vi "LUCS001RT_GPS_Processor.vi"(6 "SinchronizationReferences":T1, 7 "FPGA VI Reference Out":T3, 8 "error in":errorcluster, 11 "GPS DataIn":T4 {"UTC Valid" items=["UTC not valid", "Valid Time of Week", "Valid Week Number", "NA", "Valid UTC"]; "CAcc" format="%.0f°"; "Heading(2-D)" format="%0.6f°"; "GSpeed(2-D)" format="%.0f cm/s"; "Speed(3-D)" format="%.0f cm/s"; "NED_DNvsty" format="%.0f cm/s"; "NED_Evsty" format="%.0f cm/s"; "NED_NVsty" format="%.0f cm/s"; "Sacc" format="%.0f cm/s"; "ECEF_Z_Vlsty" format="%.0f cm/s"; "ECEF_Y_Vlsty" format="%.0f cm/s"; "ECEF_X_Vlsty" format="%.0f cm/s"; "FixType" items=["No Fix", "Dead Reckoning Only", "2D-Fix", "3D-Fix", "GPS + Dead Reckoning", "Time Only Fix", "RESERVED"]; "Vacc" format="%.0f mm"; "Hacc" format="%.0f mm"; "HMSL" format="%d mm"; "HEIGHT" format="%.0f mm"; "LAT" format="%#.6f"; "LON" format="%#.6f"; "Waypoint:XTE" format="%#.2f"}) -> (0 "error out":errorcluster, 3 "GPS Data Out":T4 {"UTC Valid" items=["UTC not valid", "Valid Time of Week", "Valid Week Number", "NA", "Valid UTC"]; "CAcc" format="%.0f°"; "Heading(2-D)" format="%0.6f°"; "GSpeed(2-D)" format="%.0f cm/s"; "Speed(3-D)" format="%.0f cm/s"; "NED_DNvsty" format="%.0f cm/s"; "NED_Evsty" format="%.0f cm/s"; "NED_NVsty" format="%.0f cm/s"; "Sacc" format="%.0f cm/s"; "ECEF_Z_Vlsty" format="%.0f cm/s"; "ECEF_Y_Vlsty" format="%.0f cm/s"; "ECEF_X_Vlsty" format="%.0f cm/s"; "FixType" items=["No Fix", "Dead Reckoning Only", "2D-Fix", "3D-Fix", "GPS + Dead Reckoning", "Time Only Fix", "RESERVED"]; "Vacc" format="%.0f mm"; "Hacc" format="%.0f mm"; "HMSL" format="%d mm"; "HEIGHT" format="%.0f mm"; "LAT" format="%#.6f"; "LON" format="%#.6f"; "Waypoint:XTE" format="%#.2f"}, 4 "GPS.DataReceived":bool)   [LabVIEW 2024]
uses:
  LUCS001RT_GPS_Data.ctl
  cRIO Projects LV8.5/UAV/TypeDefs.llb/UMV_SinchronisationReferences.ctl
panel:
  # "WAYPOINT"
  # "CURRENT POSITION"
  # "WAYPOINT"
  # "CURRENT POSITION"
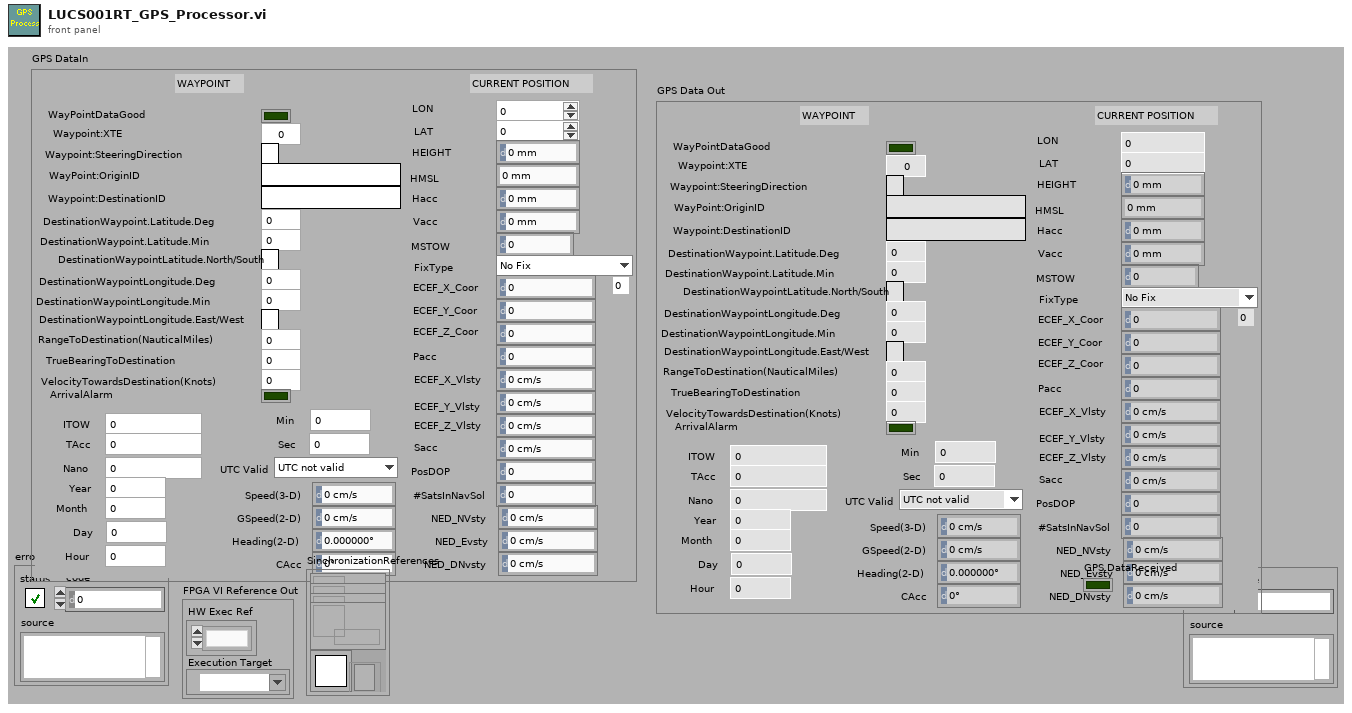
[diagram p1: front panel]
types:
  T1 = typedef "UMV_SinchronisationReferences.ctl" = cluster{"Notifier:LocalStop":refnum<notifier>, "Notifier:GlobalStop":refnum<notifier>, "RS232write":refnum<queue>, "RS232read":refnum<queue>, "RS232writeSynch":T2, "occurrence":refnum<k4>}
  T2 = typedef "Semaphore RefNum" = refnum<k1>
  T3 = cluster{"HW Exec Ref":refnum<k1>, "Execution Target":refnum<visa-resource-name>}
  T4 = typedef "LUCS001RT_GPS_Data.ctl" = cluster{"WayPointDataGood":bool, "Waypoint:XTE":dbl, "Waypoint:SteeringDirection":string, "WayPoint:OriginID":string, "Waypoint:DestinationID":string, "DestinationWaypoint.Latitude.Deg":i32, "DestinationWaypoint.Latitude.Min":dbl, "DestinationWaypointLatitude.North/South":string, "DestinationWaypointLongitude.Deg":i32, "DestinationWaypointLongitude.Min":dbl, "DestinationWaypointLongitude.East/West":string, "RangeToDestination(NauticalMiles)":dbl, "TrueBearingToDestination":dbl, "VelocityTowardsDestination(Knots)":dbl, "ArrivalAlarm":bool, "ITOW":u32, "TAcc":u32, "LON":dbl, "LAT":dbl, "HEIGHT":i32, "HMSL":i32, "Hacc":u32, "Vacc":u32, "MSTOW":u32, "FixType":u8, "ECEF_X_Coor":i32, "ECEF_Y_Coor":i32, "ECEF_Z_Coor":i32, "Pacc":u32, "ECEF_X_Vlsty":i32, "ECEF_Y_Vlsty":i32, "ECEF_Z_Vlsty":i32, "Sacc":u32, "PosDOP":u16, "#SatsInNavSol":u8, "NED_NVsty":i32, "NED_Evsty":i32, "NED_DNvsty":i32, "Speed(3-D)":u32, "GSpeed(2-D)":u32, "Heading(2-D)":dbl, "CAcc":u32, "Nano":i32, "Year":u16, "Month":u8, "Day":u8, "Hour":u8, "Min":u8, "Sec":u8, "UTC Valid":u8}
  T5 = typedef "LUCS001RT_GPS_Data.ctl" = cluster{"WayPointDataGood":bool, "Waypoint:XTE":dbl, "Waypoint:SteeringDirection":string, "WayPoint:OriginID":string, "Waypoint:DestinationID":string, "DestinationWaypoint.Latitude.Deg":i32, "DestinationWaypoint.Latitude.Min":dbl, "DestinationWaypointLatitude.North/South":string, "DestinationWaypointLongitude.Deg":i32, "DestinationWaypointLongitude.Min":dbl, "DestinationWaypointLongitude.East/West":string, "RangeToDestination(NauticalMiles)":dbl, "TrueBearingToDestination":dbl, "VelocityTowardsDestination(Knots)":dbl, "ArrivalAlarm":bool, "System.Year":dbl, "System.DayOfTehYear":dbl, "LON":dbl, "LAT":dbl, "HEIGHT":i32, "HMSL":i32, "Hacc":u32, "Vacc":u32, "MSTOW":u32, "FixType":u8, "ECEF_X_Coor":i32, "ECEF_Y_Coor":i32, "ECEF_Z_Coor":i32, "Pacc":u32, "ECEF_X_Vlsty":i32, "ECEF_Y_Vlsty":i32, "ECEF_Z_Vlsty":i32, "Sacc":u32, "PosDOP":u16, "#SatsInNavSol":u8}
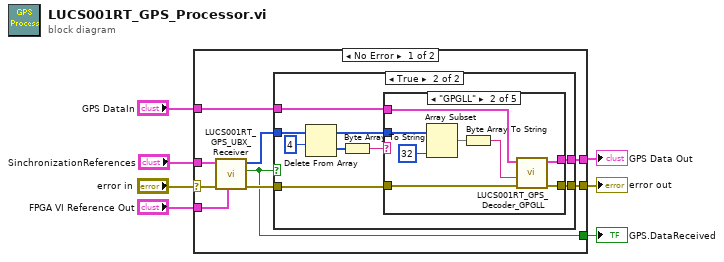
[diagram p0: block diagram]
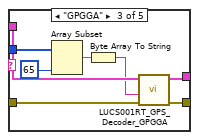
[diagram p4: hidden frame]
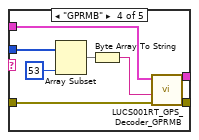
[diagram p5: hidden frame]
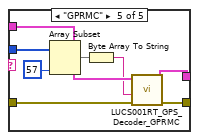
[diagram p6: hidden frame]
diagram:
  n1 = case shown="No Error" "error in" {
    selector: "error in" -> [w13 w62]
    tunnel: [w16 w62] -> w7
    tunnel: [w15 _] -> w6
    tunnel: "GPS DataIn" -> [w14 _]
    tunnel: "FPGA VI Reference Out" -> [w10 _]
    tunnel: [w9 _] -> w2
    tunnel: "SinchronizationReferences" -> [w11 _]
    frame No Error {
      n2 = call "LUCS001RT_GPS_UBX_Receiver.vi"("FPGA VI Reference In"=w10, "error in"=w13, "SinchronizationReferences"=w11) -> ("error out"=w12:errorcluster, "RX ArrayReady"=w9:bool, "GPS.TX.Message"=w8:u8[])  [unwired: 6 in]
      n3 = case shown="True" w9 {
        tunnel: [w18 w27] -> w16
        tunnel: [w17 w26] -> w15
        tunnel: w14 -> [w17 w25]
        tunnel: w12 -> [w18 w24]
        tunnel: w8 -> [_ w20]
        frame False {
        }
        frame True {
          n4 = Delete From Array(array=w20, length=4) -> (deleted portion=w19:u8[], array with subset deleted=w21:u8[])  [unwired: 1 in]
          n5 = Byte Array To String(unsigned byte array=w19) -> (string=w22:string)
          n6 = case shown="\"GPGLL\"" w22 {
            tunnel: w24 -> [w29 w33 w40 w50 w58]
            tunnel: [w29 w35 w43 w53 w61] -> w27
            tunnel: w25 -> [w28 w37 w45 w52 w60]
            tunnel: [w28 w36 w44 w51 w59] -> w26
            tunnel: w21 -> [_ w31 w39 w47 w55]
            frame Default {
            }
            frame "GPGLL" {
              n7 = Array Subset(array=w31, length=32 ("byte count")) -> (w30:u8[])  [unwired: 1 in]
              n8 = Byte Array To String(unsigned byte array=w30) -> (string=w32:string)
              n9 = call "LUCS001RT_GPS_Decoder_GPGLL.vi"("error in (no error)"=w33, "SerialData: GPGLL"=w32, "GPS Data In"=w37) -> ("error out"=w35:errorcluster, "GPS Data Out"=w36:T4)  [unwired: 7 in]
            }
            frame "GPGGA" {
              n10 = Array Subset(array=w39, length=65 ("byte count")) -> (w38:u8[])  [unwired: 1 in]
              n11 = Byte Array To String(unsigned byte array=w38) -> (string=w41:string)
              n12 = call "LUCS001RT_GPS_Decoder_GPGGA.vi"("error in (no error)"=w40, "SerialData: GPGLL"=w41, "GPS Data In"=w45) -> ("error out"=w43:errorcluster, "GPS Data Out"=w44:T4)  [unwired: 7 in]
            }
            frame "GPRMB" {
              n13 = Array Subset(array=w47, length=53 ("byte count")) -> (w46:u8[])  [unwired: 1 in]
              n14 = Byte Array To String(unsigned byte array=w46) -> (string=w48:string)
              n15 = call "LUCS001RT_GPS_Decoder_GPRMB.vi"("error in (no error)"=w50, "SerialData:$GPRMB"=w48, "GPS DataIn"=w52) -> ("error out"=w53:errorcluster, "GPS DataOut"=w51:T4)  [unwired: 7 in]
            }
            frame "GPRMC" {
              n16 = Array Subset(array=w55, length=57 ("byte count")) -> (w54:u8[])  [unwired: 1 in]
              n17 = Byte Array To String(unsigned byte array=w54) -> (string=w56:string)
              n18 = call "LUCS001RT_GPS_Decoder_GPRMC.vi"("error in"=w58, "SerialData"=w56, "GPS Data"=w60) -> ("error out"=w61:errorcluster, "GPS Data Out"=w59:T5)  [unwired: 7 in]
            }
          }
        }
      }
    }
    frame Error {
    }
  }
  "error out" <- w7
  "GPS Data Out" <- w6
  "GPS.DataReceived" <- w2
